vi "_Append Variable Source File in Map.vi"(7 "String":string, 8 "error in (no error)":errorcluster, 9 "dup path":path, 10 "Content":string, 11 "Variable-FileMap":variant) -> (0 "error out":errorcluster, 3 "Variant":variant)   [LabVIEW 2017, in "INI-Static-Variable-Support.lvlib" / "CSM-Static-Variable-Manager.lvclass"]
uses:
  CSM-Static-Variable-Manager.lvclass
  <userlib>/_NEVSTOP/Communicable State Machine(CSM)/addons/API-String-Arugments-Support/API String Arguments Support.lvlib
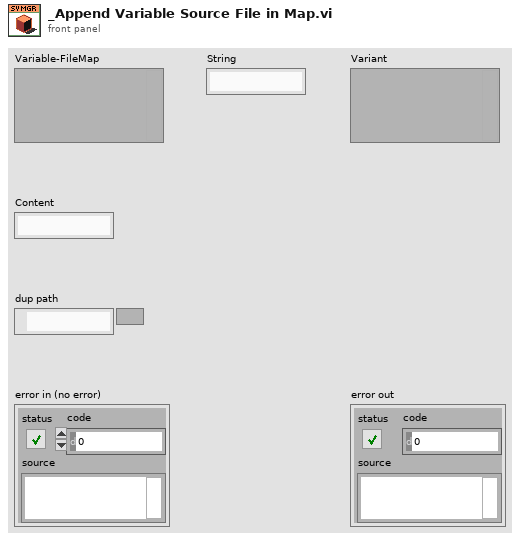
[diagram p1: front panel]
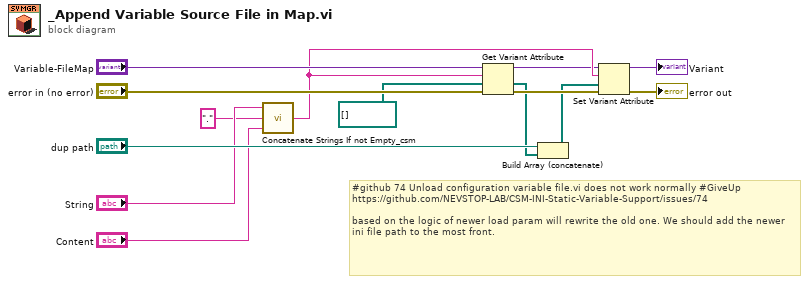
[diagram p0: block diagram]
diagram:
  # "#github 74 Unload configuration variable file.vi does not work normally #GiveUp\nhttps://github.com/NEVSTOP-LAB/CSM-INI-Static-Variable-Support/issues/74\n\nbased on the logic of newer load param will rewrite the old one. We should add the newer ini file path to the most front."
  n1 = call <userlib>:"Concatenate Strings If not Empty_csm.vi"("String"="Content", "seperator(:)"=".", "prefix"="String") -> ("result"=w9:string)  [unwired: 2 in]
  n2 = Get Variant Attribute(Variant="Variable-FileMap", name=w9, default value (empty Variant)=path[] [], error in="error in (no error)") -> (duplicate Variant=w7:variant, value=w5:path[], error out=w10:errorcluster)  [unwired: 1 out]
  n3 = Build Array (concatenate)("dup path", w5) -> (w8:path[])
  n4 = Set Variant Attribute(Variant=w7, name=w9, value=w8, error in=w10) -> (Variant out=→"Variant":variant, error out=→"error out":errorcluster)  [unwired: 1 out]
